vi "transform MessageProperties.vi"(11 "properties (KVP)":variant) -> (3 "properties (Variant Attr)":variant)   [LabVIEW 2020, in "Caraya.lvlib" / "Test Event Storage.lvclass"]
uses:
  Test Event Storage.lvclass
  Test Manager Message KVP/TestManagerMsg.KVP.lvclass
  C:/projects/caraya/src/classes/Test Manager Message/TestManagerMsg.lvclass
  Test Manager Message KVP/TestManagerMsg.KVP.lvclass/TestManagerMsg.KVP.ctl
  Test Manager Message/TestManagerMsg.lvclass/TestManagerMsg.ctl
  Test Manager Message/TestManagerMsg.lvclass
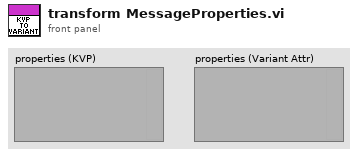
[diagram p1: front panel]
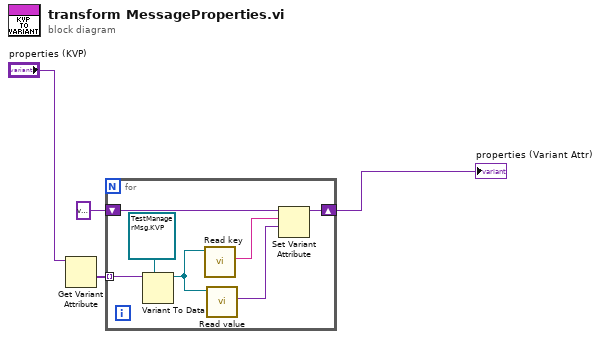
[diagram p0: block diagram]
diagram:
  n1 = Get Variant Attribute(Variant="properties (KVP)") -> (values=w1:variant[])  [unwired: 3 in, 3 out]
  n2 = for {
    tunnel: w1 -> [w11] mode=indexing
    shift-right: [w8] -> w4
    shift-left: variant ("properties") -> [w7]
    n3 = Variant To Data(type=refnum<class "TestManagerMsg.KVP.lvclass"> refnum ("Caraya.lvlib:TestManagerMsg.KVP.lvclass"), Variant=w11) -> (data=w9:refnum<class "TestManagerMsg.KVP.lvclass">)  [unwired: 1 in, 1 out]
    n4 = call "Read key.vi"("TestManagerMsg in"=w9) -> ("key"=w6:string)  [unwired: 9 in, 1 out]
    n5 = call "Read value.vi"("TestManagerMsg.KVP in"=w9) -> ("value"=w5:variant)  [unwired: 9 in, 1 out]
    n6 = Set Variant Attribute(Variant=w7, name=w6, value=w5) -> (Variant out=w8:variant)  [unwired: 1 in, 2 out]
  }
  "properties (Variant Attr)" <- w4
